vi "init.vi"(0 "Digital Output Test in":refnum<class "Digital Output Test.lvclass">, 1 "DAQ Channel to Read":refnum<k21>, 2 "Value to Test":u16, 3 "Value to Expect":T1, 4 "ConfigureILCStrategy":refnum<class "IConfigureILCStrategy.lvclass">, 5 "error in (no error)":errorcluster, 6 "Test Scenario":T2, 7 "ILC":refnum<class "ILC.lvclass">, 8 "Signal Name":string, 9 "Log":refnum<class "ITestLog.lvclass">) -> (14 "Digital Output Test out":refnum<class "Digital Output Test.lvclass">, 19 "error out":errorcluster)   [LabVIEW 2015, in "Digital Output Test.lvclass"]
uses:
  Digital Output Test.lvclass
  Model/TestLog/ITestLog/ITestLog.lvclass
  Typedefs/TestScenarioTypes.ctl
  Model/ConfigureILCStrategy/IConfigureILCStrategy/IConfigureILCStrategy.lvclass
  <userlib>/Common/ilc/ILC/ILC.lvclass
  Typedefs/Digital Signal Level.ctl
  Digital Output Test.lvclass/Digital Output Test.ctl
  Typedefs/ILCBTTypedefs.lvlib
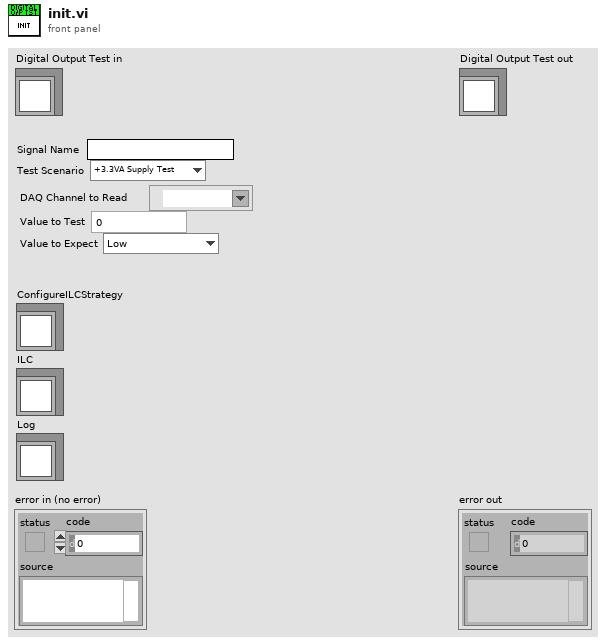
[diagram p1: front panel]
types:
  T1 = typedef "ILCBTTypedefs.lvlib/Digital Signal Level.ctl" = enum16{"Low", "High"}
  T2 = typedef "ILCBTTypedefs.lvlib/TestScenarioTypes.ctl" = enum16{"+3.3VA Supply Test", "+3.3VD Supply Test", "+5VA Supply Test", "+5VD Supply Test", "Unique ID Test", "TEDS Status Test", "LIMSW1_TTL Low Test", "LIMSW1_TTL High Test", "LIMSW2_TTL Low Test", "LIMSW2_TTL High Test", "Tachometer Test", "SSR_TTL Low Test", "SSR_TTL High Test", "SM_CW Low Test", "SM_CW High Test", "SM_CCW Low Test", "SM_CCW High Test", "SM_GPI Low Test", "SM_GPI High Test", "CW Motion Without Limit Test", "CW Motion With Limit Test", "CW Motion With Limit Interruption Test", "CW Motion on CCW Limit Test", "CCW Motion Without Limit Test", "CCW Motion With Limit Test", "CCW Motion With Limit Interruption Test", "CCW Motion on CW Limit Test", "RS232-TXD Low Test", "RS232-TXD High Test", "RS232-RTS Low Test", "RS232-RTS High Test", "RS232-RXD Low Test", "RS232-RXD High Test", "RS232-CTS Low Test", "RS232-CTS High Test", "Out_SS Low Test", "Out_SS High Test", "Out_SDI Low Test", "Out_SDI High Test", "Out_SCLK Low Test", "Out_SCLK High Test", "Reset Low Test", "Reset High Test", "1 Channel ADC Test", "3 Channel ADC Test", "5 Channel ADC Test", "Vref Test", "ROT Test", "DAC1 Test", "DAC2 Test", "DAC3 Test", "DAC4 Test", "BIAS Test", "EXC1 Test", "EXC2 Test", "EXC3 Test", "EXC4 Test"}
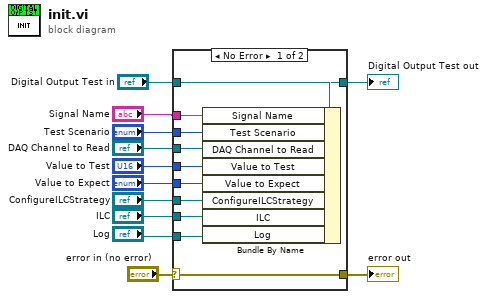
[diagram p0: block diagram]
diagram:
  n1 = case shown="No Error" "error in (no error)" {
    selector: "error in (no error)" -> [w23 w25]
    tunnel: [w23 w25] -> w11
    tunnel: [w13 w24] -> w9
    tunnel: "Digital Output Test in" -> [w22 w24]
    tunnel: "Signal Name" -> [w21 _]
    tunnel: "Test Scenario" -> [w20 _]
    tunnel: "ConfigureILCStrategy" -> [w16 _]
    tunnel: "ILC" -> [w17 _]
    tunnel: "Log" -> [w18 _]
    tunnel: "DAQ Channel to Read" -> [w19 _]
    tunnel: "Value to Test" -> [w15 _]
    tunnel: "Value to Expect" -> [w14 _]
    frame No Error {
      n2 = Bundle By Name(cluster=w22, "Signal Name"=w21, "Test Scenario"=w20, "DAQ Channel to Read"=w19, "Value to Test"=w15, "Value to Expect"=w14, "ConfigureILCStrategy"=w16, "ILC"=w17, "Log"=w18) -> (w13:refnum<class "Digital Output Test.lvclass">)
    }
    frame Error {
    }
  }
  "error out" <- w11
  "Digital Output Test out" <- w9
